vi "Read Sum.vi"(11 "TestActor in":refnum<class "TestActor.lvclass">) -> (2 "Sum":dbl, 3 "TestActor out":refnum<class "TestActor.lvclass">)   [LabVIEW 2020, in "Messaging Tests.lvlib" / "TestActor.lvclass"]
uses:
  TestActor.lvclass
  TestActor.lvclass/TestActor.ctl
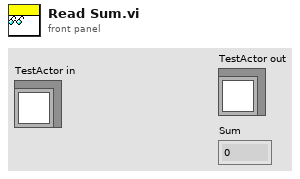
[diagram p1: front panel]
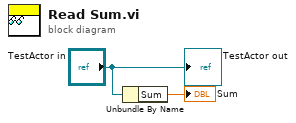
[diagram p0: block diagram]
diagram:
  n1 = Unbundle By Name("TestActor in") -> ("Sum"=→"Sum":dbl)
  "TestActor out" <- "TestActor in"
